vi "Target - REF3 - MAIN.vi"() -> ()   [LabVIEW 2013]
doc: "This VI first configures the sample clock on the module and starts it. Then it acquires single point data from four channels. In order for the loop rate to be synchronized with the module's clock, the data is pipelined before it is written it to a DMA FIFO so it can be transfered to the host."
uses:
  <vilib>/LabVIEW Targets/FPGA/cRIO/shared/nicrio_ModuleControls/nicrio_cRIO-9234_DataRatesRing2.ctl
  <vilib>/rvi/eio/common/nirviEmuTemplatePropertySet_errors.vi
  <vilib>/rvi/eio/common/nirviEmuTemplateMethod_errors.vi
  <vilib>/rvi/Emulation/niFpgaSctlEmulationGetInTimedLoop.vi
  <vilib>/rvi/Emulation/niFpgaEmulationReportErrorSimple.vi
  <vilib>/rvi/Emulation/niFpgaGetClockAttributes.vi
  <vilib>/rvi/Emulation/niFpgaCriticalErrorInLSC.vi
  <vilib>/rvi/eio/common/nirviEmuTemplatePropertyGet_noerrors.vi
  <vilib>/rvi/interface/RandomDataEmulation/nirviRandomDataFPGAFIFO.vi
  <vilib>/rvi/interface/RandomDataEmulation/niFpgaRandomDataHandleErrors.vi
  <vilib>/eio/EIOPropertyNode/EIOPropertyNode.xnode
  <vilib>/eio/EIONode/EIONode.xnode
  <vilib>/eio/EIOMethodNode/EIOMethodNode.xnode
  <vilib>/rvi/DataTransferAndStorage/Container/XNode/niFpgaContainer.xnode
  <vilib>/rvi/interface/RandomDataEmulation/nirviRandomDataFpgaReadWriteTemplate.vi
  <vilib>/rvi/eio/common/nirviEmuTemplatePropertyGet_errors.vi
  <vilib>/rvi/eio/common/nirviEmuTemplatePropertySet_noerrors.vi
  GPS Timekeeper Files/FPGA Timekeeper.lvlib
panel:
  out "FPGA Timekeeper time (ns)":u64
  out "GPS status":T1(ring)
  out "FPGA Timekeeper locked":bool
  out "offset from time reference":i32
  out "antenna status":T2(ring)
  out "satellites available":u8
  out "UTC offset":i8
  out "UTC offset valid":bool
  in  "Data Rate":T3=1 items=["51.200 kS/s (NI 9234)"=1, "25.600 kS/s (NI 9234)"=2, "17.067 kS/s (NI 9234)"=3, "12.800 kS/s (NI 9234)"=4, "10.240 kS/s (NI 9234)"=5, "8.533 kS/s (NI 9234)"=6, "7.314 kS/s (NI 9234)"=7, "6.400 kS/s (NI 9234)"=8, "5.689 kS/s (NI 9234)"=9, "5.120 kS/s (NI 9234)"=10, "4.654 kS/s (NI 9234)"=11, "4.267 kS/s (NI 9234)"=12, "3.938 kS/s (NI 9234)"=13, "3.657 kS/s (NI 9234)"=14, "3.413 kS/s (NI 9234)"=15, "3.200 kS/s (NI 9234)"=16, "3.012 kS/s (NI 9234)"=17, "2.845 kS/s (NI 9234)"=18, "2.695 kS/s (NI 9234)"=19, "2.560 kS/s (NI 9234)"=20, "2.438 kS/s (NI 9234)"=21, "2.328 kS/s (NI 9234)"=22, "2.226 kS/s (NI 9234)"=23, "2.133 kS/s (NI 9234)"=24, "2.048 kS/s (NI 9234)"=25, "1.969 kS/s (NI 9234)"=26, "1.896 kS/s (NI 9234)"=27, "1.829 kS/s (NI 9234)"=28, "1.765 kS/s (NI 9234)"=29, "1.707 kS/s (NI 9234)"=30, "1.652 kS/s (NI 9234)"=31]
  out "Acq Loop Ticks":u32
  out "FPGA Error":errorcluster
  out "Module Underflow":bool
  out "DMA FIFO Full":bool
  in  "Stop":bool
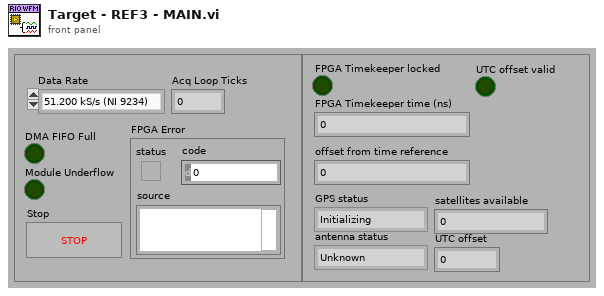
[diagram p1: front panel]
types:
  T1 = enum8{"Initializing", "Normal", "Unable to get fix"}
  T2 = enum8{"Unknown", "Normal", "Absent", "Overcurrent"}
  T3 = typedef "nicrio_cRIO-9234_DataRatesRing2.ctl" = u8
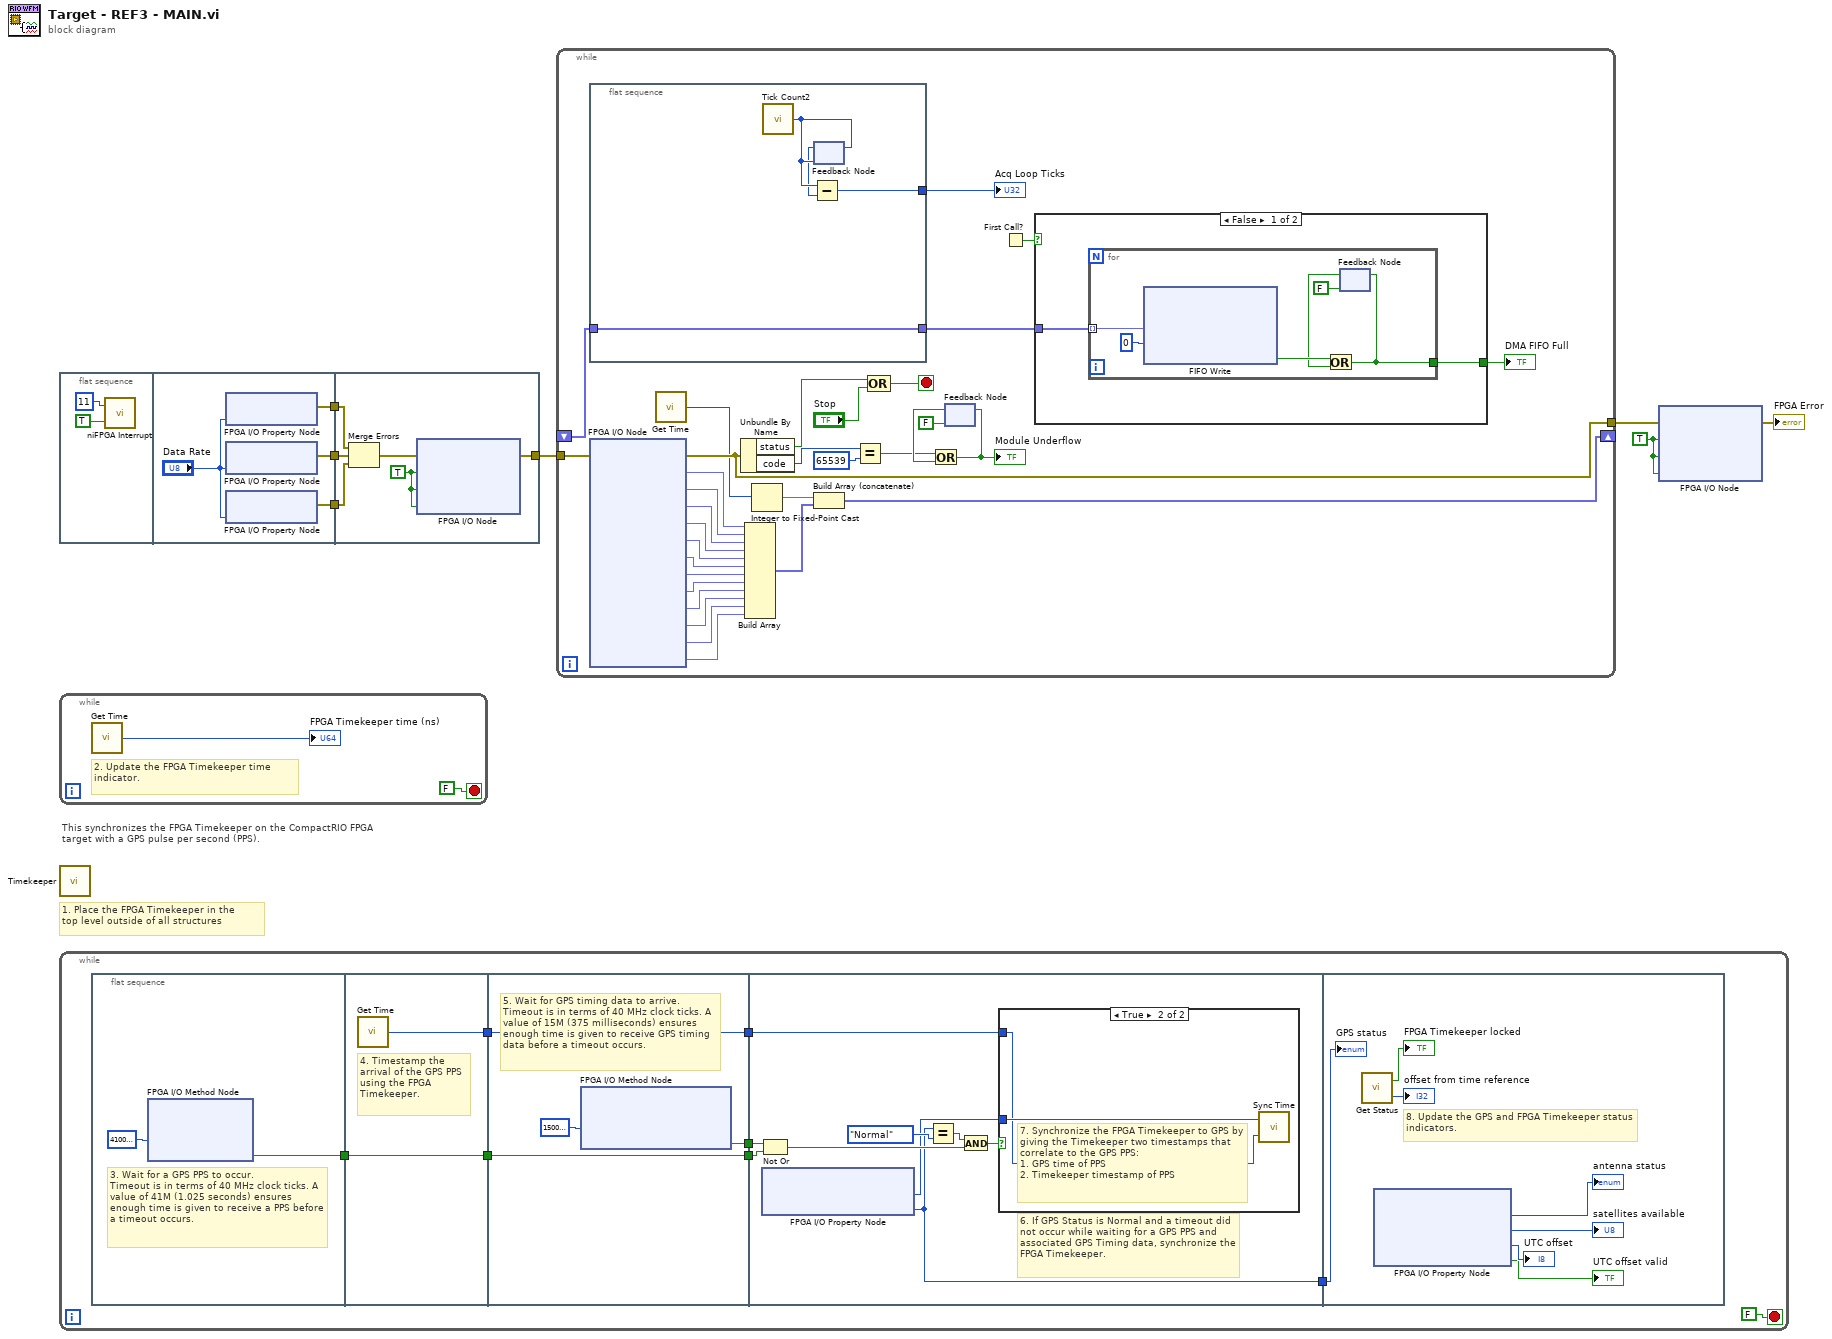
[diagram p0: block diagram]
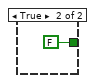
[diagram p3: hidden frame]
diagram:
  w1 = TRUE ("Mod1/Stop")
  # "This synchronizes the FPGA Timekeeper on the CompactRIO FPGA target with a GPS pulse per second (PPS)."
  # "1. Place the FPGA Timekeeper in the\ntop level outside of all structures"
  n1 = flat-sequence {
    tunnel: [w13] -> w6
    tunnel: [w12] -> w3
    tunnel: [w10] -> w2
    tunnel: [w19] -> w7
    tunnel: w6 -> [w17]
    tunnel: w3 -> [w16]
    tunnel: w2 -> [w15]
    frame #0 {
      n2 = call <vilib>:"niFPGA Interrupt.vi"("Wait Until Cleared (F)"=TRUE ("Wait Until Cleared"), "IRQ Number (0)"=u8 11 ("IRQ Number")) -> ()  [unwired: 1 in]
    }
    frame #1 {
      n3 = xnode "FPGA I/O Property Node"("Data Rate"="Data Rate") -> ("error out"=w10:errorcluster)  [unwired: 2 in, 1 out]
      n4 = xnode "FPGA I/O Property Node"("Data Rate"="Data Rate") -> ("error out"=w13:errorcluster)  [unwired: 2 in, 1 out]
      n5 = xnode "FPGA I/O Property Node"("Data Rate"="Data Rate") -> ("error out"=w12:errorcluster)  [unwired: 2 in, 1 out]
    }
    frame #2 {
      w14 = TRUE ("Mod1/Start")
      n6 = Merge Errors(w15, w17, w16) -> (w18:errorcluster)
      n7 = xnode "FPGA I/O Node"("error in"=w18, "Mod5/Start"=w14, "Mod6/Start"=w14, "Mod7/Start"=w14) -> ("error out"=w19:errorcluster)  [unwired: 3 in, 3 out]
    }
  }
  n8 = while {
    stop <- FALSE stop-if-true
    # "2. Update the FPGA Timekeeper time indicator."
    n9 = call "Get Time.vi"() -> ("time (ns)"=→"FPGA Timekeeper time (ns)":u64)  [unwired: 1 in]
  }
  n10 = call "Timekeeper.vi"() -> ()  [unwired: 12 in]
  n11 = while {
    stop <- FALSE stop-if-true
    n12 = flat-sequence {
      tunnel: [w30] -> w28
      tunnel: w28 -> [w33]
      tunnel: [w33] -> w27
      tunnel: [w32] -> w25
      tunnel: [w36] -> w29
      tunnel: w27 -> [w35]
      tunnel: [w35] -> w26
      tunnel: w25 -> [w34]
      tunnel: [w34] -> w24
      tunnel: w29 -> [w45]
      tunnel: w26 -> [w44]
      tunnel: w24 -> [w39]
      tunnel: [w38] -> w23
      tunnel: w23 -> [w55]
      frame #0 {
        # "3. Wait for a GPS PPS to occur.\nTimeout is in terms of 40 MHz clock ticks. A value of 41M (1.025 seconds) ensures enough time is given to receive a PPS before a timeout occurs."
        n13 = xnode "FPGA I/O Method Node"("Timeout"=41000000) -> ("Timed Out"=w30:bool)  [unwired: 1 in, 1 out]
      }
      frame #1 {
        # "4. Timestamp the arrival of the GPS PPS using the FPGA Timekeeper."
        n14 = call "Get Time.vi"() -> ("time (ns)"=w32:u64)  [unwired: 1 in]
      }
      frame #2 {
        # "5. Wait for GPS timing data to arrive.\nTimeout is in terms of 40 MHz clock ticks. A value of 15M (375 milliseconds) ensures enough time is given to receive GPS timing data before a timeout occurs."
        n15 = xnode "FPGA I/O Method Node"("Timeout"=15000000) -> ("Timed Out"=w36:bool)  [unwired: 1 in, 1 out]
      }
      frame #3 {
        # "6. If GPS Status is Normal and a timeout did not occur while waiting for a GPS PPS and associated GPS Timing data, synchronize the FPGA Timekeeper."
        n16 = Not Or(1:w44, 2:w45) -> (0:w42:bool)
        n17 = xnode "FPGA I/O Property Node"() -> ("PPS Timestamp (TAI)"=w40:u64, "GPS Status"=w38:T1)  [unwired: 1 in, 1 out]
        n18 = Equal?(x=w38, y=T1."Normal") -> (x = y?=w43:bool)
        n19 = And(x=w43, y=w42) -> (x .and. y?=w41:bool)
        n20 = case shown="True" w41 {
          tunnel: w40 -> [_ w48]
          tunnel: w39 -> [_ w47]
          frame False {
          }
          frame True {
            # "7. Synchronize the FPGA Timekeeper to GPS by giving the Timekeeper two timestamps that correlate to the GPS PPS:\n1. GPS time of PPS\n2. Timekeeper timestamp of PPS"
            n21 = call "Sync Time.vi"("FPGA Timekeeper time (ns)"=w47, "time reference time (ns)"=w48) -> ()
          }
        }
      }
      frame #4 {
        # "8. Update the GPS and FPGA Timekeeper status indicators."
        n22 = call "Get Status.vi"() -> ("FPGA Timekeeper locked"=→"FPGA Timekeeper locked":bool, "offset from time reference"=→"offset from time reference":i32)
        n23 = xnode "FPGA I/O Property Node"() -> ("Antenna Status"=→"antenna status":T2, "Satellites Available"=→"satellites available":u8, "UTC Offset"=→"UTC offset":i8, "UTC Offset Valid"=→"UTC offset valid":bool)  [unwired: 1 in, 1 out]
        "GPS status" <- w55
      }
    }
  }
  n24 = while {
    tunnel: [w83] -> w5
    shift-right: [w71] -> _
    shift-left: _ -> [w79]
    tunnel: w7 -> [w72]
    stop <- w86 stop-if-true
    n25 = flat-sequence {
      tunnel: [w98] -> w81
      tunnel: w79 -> [w97]
      tunnel: [w97] -> w80
      frame #0 {
        n26 = call "Tick Count2"() -> ("Tick Count(Ticks)"=w100:u32)
        n27 = feedback-in #1(w100) -> ()
        n28 = feedback #1(w100) -> (w99:u32)
        n29 = Subtract(x=w100, y=w99) -> (x-y=w98:u32)
      }
    }
    n30 = xnode "FPGA I/O Node"("error in"=w72) -> ("error out"=w83:errorcluster, "Mod5/AI0"=w56:fxp<+/-,24,4>, "Mod5/AI1"=w57:fxp<+/-,24,4>, "Mod5/AI2"=w58:fxp<+/-,24,4>, "Mod5/AI3"=w59:fxp<+/-,24,4>, "Mod6/AI0"=w68:fxp<+/-,24,4>, "Mod6/AI1"=w67:fxp<+/-,24,4>, "Mod6/AI2"=w66:fxp<+/-,24,4>, "Mod6/AI3"=w65:fxp<+/-,24,4>, "Mod7/AI0"=w63:fxp<+/-,24,4>, "Mod7/AI1"=w62:fxp<+/-,24,4>, "Mod7/AI2"=w61:fxp<+/-,24,4>, "Mod7/AI3"=w60:fxp<+/-,24,4>)  [unwired: 12 in, 12 out]
    n31 = call "Get Time.vi"() -> ("time (ns)"=w64:u64)  [unwired: 1 in]
    n32 = Unbundle By Name(w83) -> ("status"=w78:bool, "code"=w84:i32)
    n33 = Build Array(w56, w57, w58, w59, w68, w67, w66, w65, w63, w62, w61, w60) -> (w69:fxp<+/-,24,4>[])
    n34 = Integer to Fixed-Point Cast(integer=w64) -> (fixed-point=w70:fxp<+/-,64,44>)  [unwired: 1 in]
    n35 = Build Array (concatenate)(w70, w69) -> (w71:fxp<+/-,64,44>[])
    n36 = Equal?(x=w84, y=65539) -> (x = y?=w75:bool)
    n37 = Compound Arithmetic op=OR(w78, "Stop") -> (w86:bool)
    n38 = feedback #2(FALSE) -> (w77:bool)
    n39 = Or(x=w75, y=w77) -> (x .or. y?=w74:bool)
    "Module Underflow" <- w74
    n40 = feedback-in #2(w74) -> ()
    n41 = First Call?() -> (First Call?: T/F=w73:bool)
    n42 = case shown="False" w73 {
      tunnel: [w89 FALSE] -> w82
      tunnel: w80 -> [w88 _]
      frame False {
        n43 = for {
          tunnel: [w92] -> w89
          tunnel: w88 -> [w90] mode=indexing
          n44 = xnode ("FIFO Write")("Element"=w90, "Timeout"=0) -> ("Timed Out?"=w95:bool)  [unwired: 1 in, 1 out]
          n45 = feedback #3(FALSE) -> (w93:bool)
          n46 = Or(x=w95, y=w93) -> (x .or. y?=w92:bool)
          n47 = feedback-in #3(w92) -> ()
        }
      }
      frame True {
      }
    }
    "DMA FIFO Full" <- w82
    "Acq Loop Ticks" <- w81
  }
  n48 = xnode "FPGA I/O Node"("error in"=w5, "Mod5/Stop"=w1, "Mod6/Stop"=w1, "Mod7/Stop"=w1) -> ("error out"=→"FPGA Error":errorcluster)  [unwired: 3 in, 3 out]
